vi "ControlKeithley2614_B.vi"() -> ()   [LabVIEW 2015]
panel:
  in  "GPIB Address":string="12"
  out "String":string
  in  "Record new values":bool
  out "Output Current (A)":dbl
  out "Output Voltage (V)":dbl
  out "Compliance limit (V)":dbl
  out "Current Range":u16(ring) items=["100 nA", "1 uA", "10 uA", "100 uA", "1 mA", "10 mA", "100 mA", "1 A"]
  out "Voltage Range":u16(ring) items=["200 mV", "2 V", "20 V", "200 V"]
  out "Current (sourse)":dbl
  out "Voltage (sourse)":dbl
  out "ComplianceIndicator":bool
  out "Compliance limit (A)":dbl
  out "Source Function":u16(ring)=1 items=["Current Source", "Voltage Source"]
  out "Sence Mode":u16(ring) items=["2-wire", "4-wire"]
  in  "ON/OFF channel":bool
  out "ON/OFF indicator":bool
  in  "error in (no error)":errorcluster
  out "error out":errorcluster
  # "Channel B"
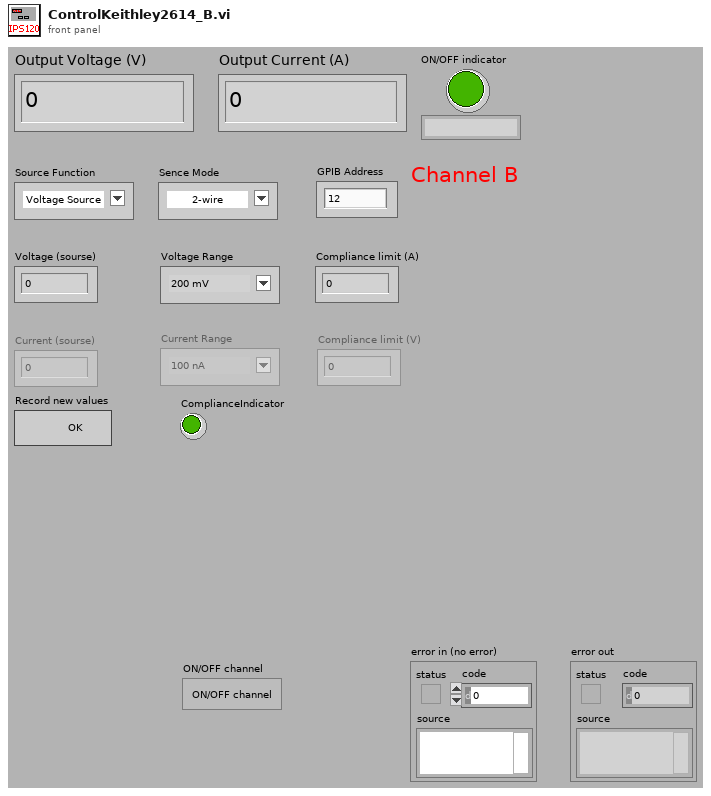
[diagram p1: front panel]
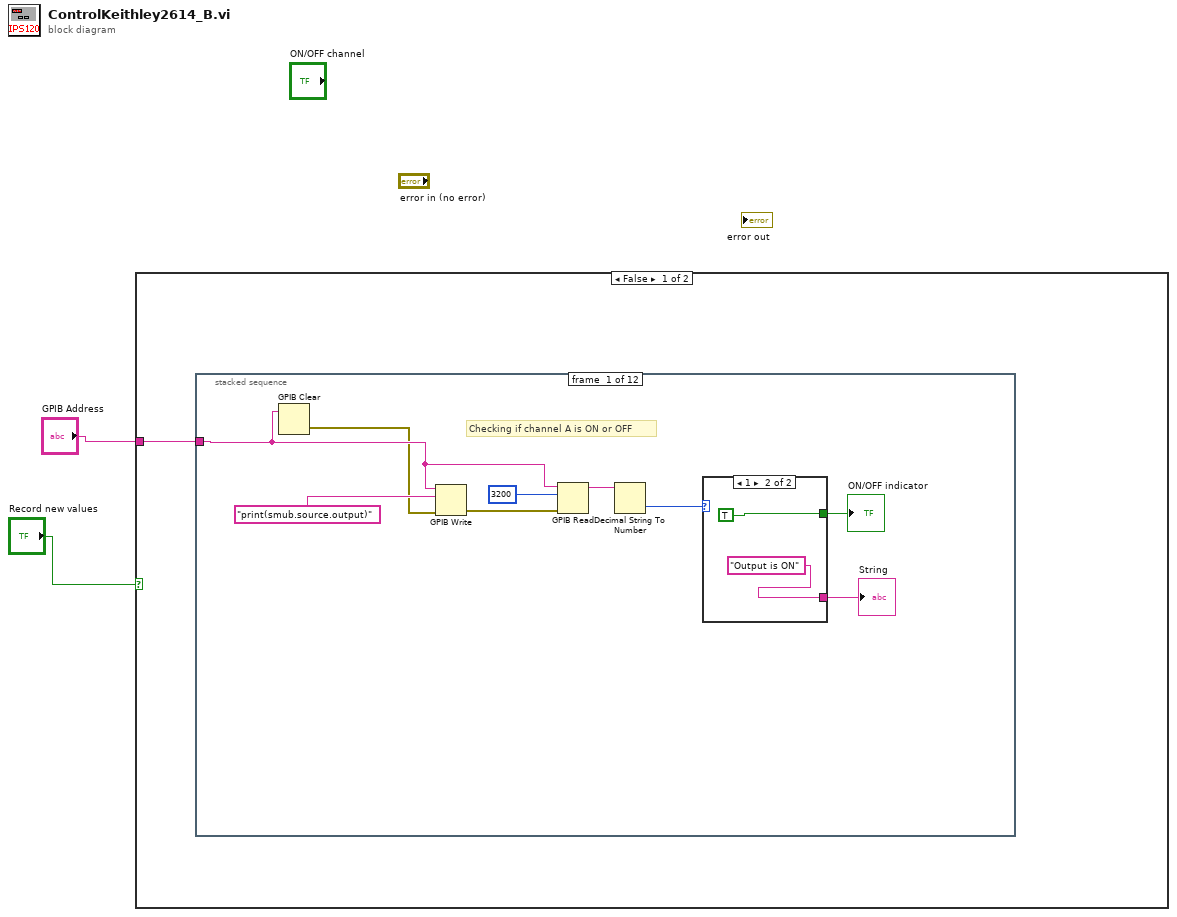
[diagram p0: block diagram]
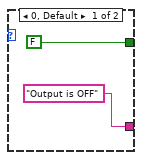
[diagram p2: hidden frame]
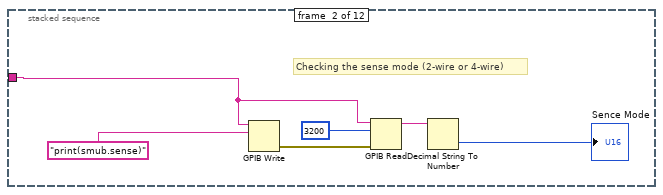
[diagram p3: hidden frame]
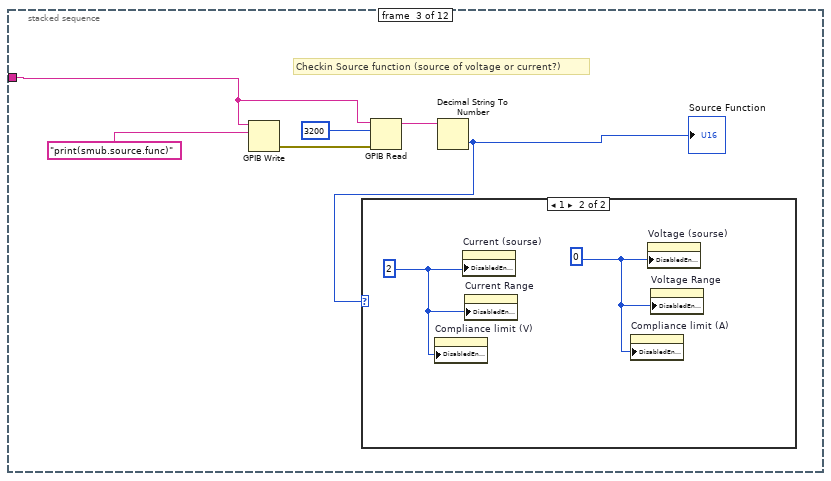
[diagram p4: hidden frame]
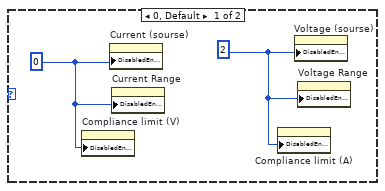
[diagram p5: hidden frame]
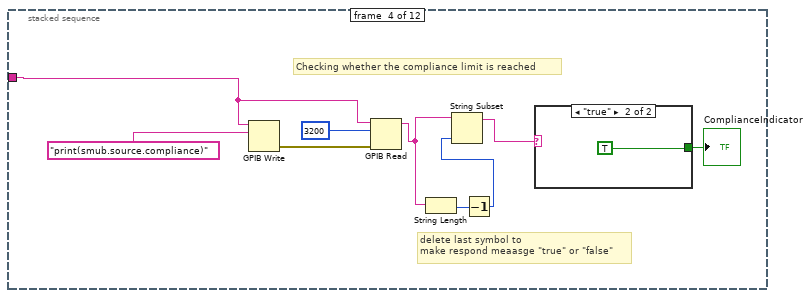
[diagram p6: hidden frame]
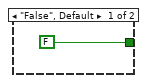
[diagram p7: hidden frame]
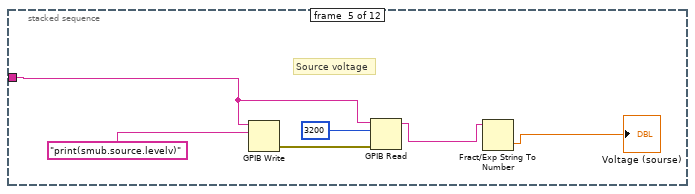
[diagram p8: hidden frame]
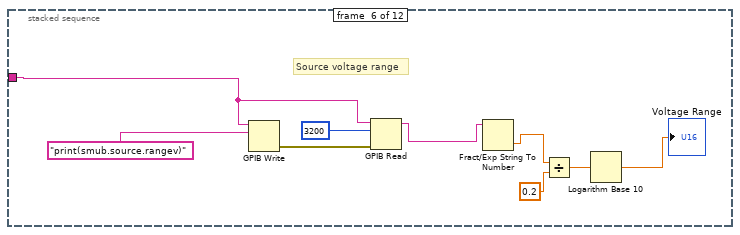
[diagram p9: hidden frame]
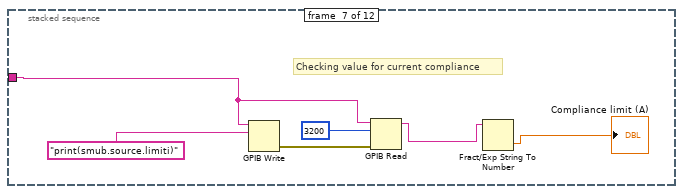
[diagram p10: hidden frame]
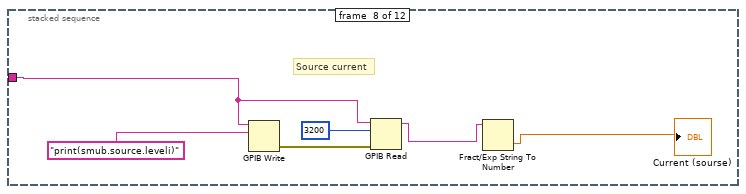
[diagram p11: hidden frame]
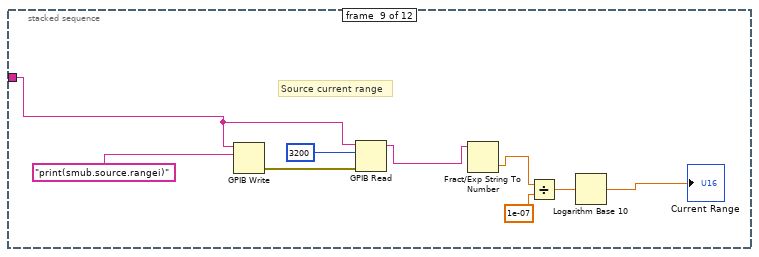
[diagram p12: hidden frame]
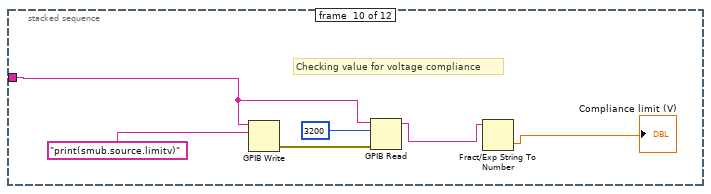
[diagram p13: hidden frame]
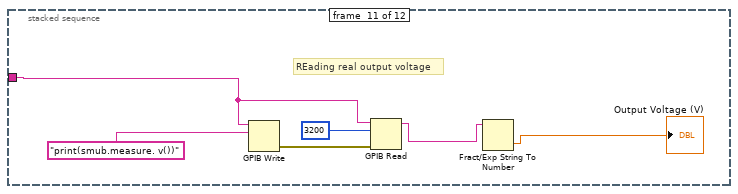
[diagram p14: hidden frame]
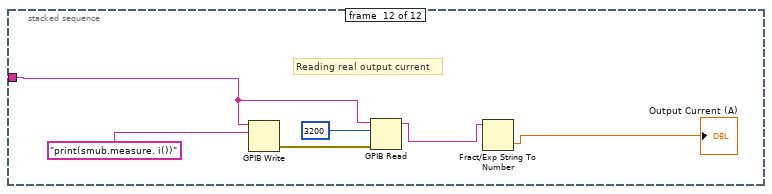
[diagram p15: hidden frame]
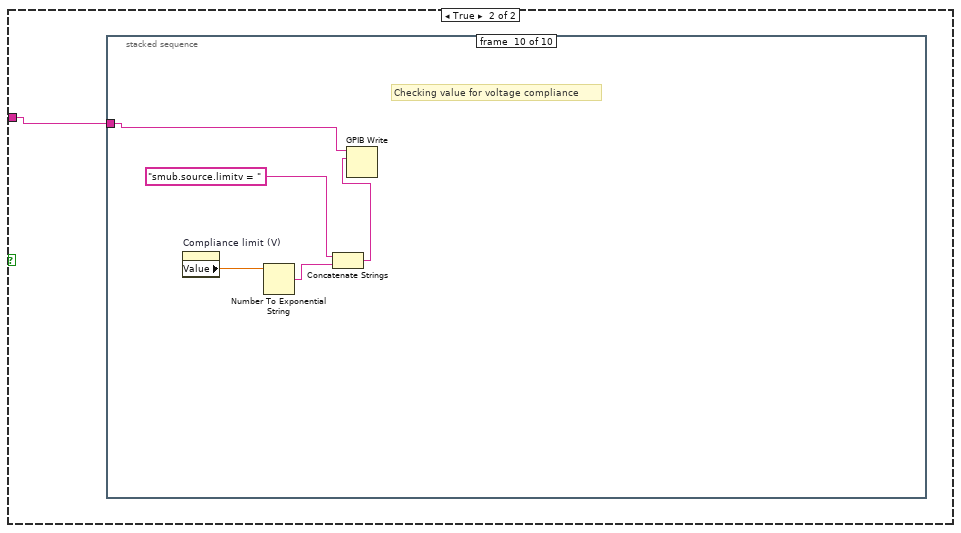
[diagram p16: hidden frame]
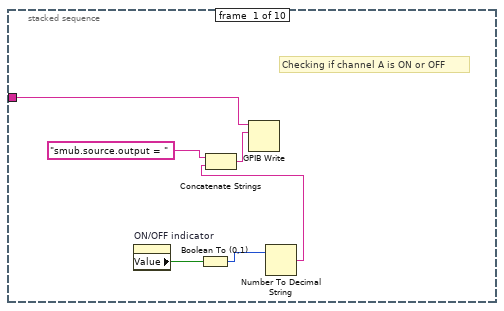
[diagram p17: hidden frame]
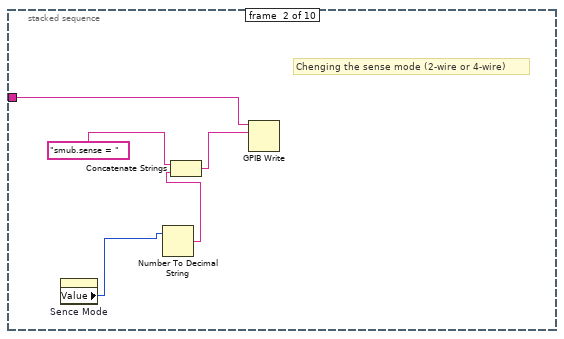
[diagram p18: hidden frame]
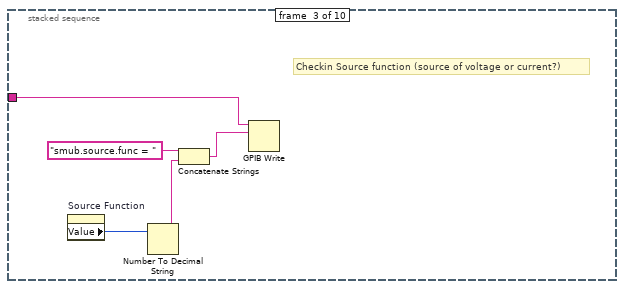
[diagram p19: hidden frame]
diagram:
  n1 = case shown="False" "Record new values" {
    tunnel: "GPIB Address" -> [w3 w98]
    frame False {
      n2 = stacked-sequence {
        tunnel: w3 -> [w5 w17 w23 w33 w44 w50 w59 w65 w71 w80 w86 w92]
        frame #0 {
          # "Checking if channel A is ON or OFF"
          n3 = GPIB Clear(3:w5) -> (0:w4:errorcluster)  [unwired: 1 in, 1 out]
          n4 = GPIB Write(0:w5, 1:"print(smub.source.output)", 3:w4) -> (6:w12:errorcluster)  [unwired: 2 in, 1 out]
          n5 = GPIB Read(0:w5, 1:3200, 3:w12) -> (5:w9:string)  [unwired: 2 in, 2 out]
          n6 = Decimal String To Number(string=w9) -> (number=w8:i32)  [unwired: 2 in, 1 out]
          n7 = case shown="1" w8 {
            tunnel: [FALSE TRUE] -> w7
            tunnel: ["Output is OFF" "Output is ON"] -> w6
            frame 0, Default {
            }
            frame 1 {
            }
          }
          "ON/OFF indicator" <- w7
          "String" <- w6
        }
        frame #1 {
          # "Checking the sense mode (2-wire or 4-wire)"
          n8 = GPIB Write(0:w17, 1:"print(smub.sense)") -> (6:w22:errorcluster)  [unwired: 3 in, 1 out]
          n9 = GPIB Read(0:w17, 1:3200, 3:w22) -> (5:w19:string)  [unwired: 2 in, 2 out]
          n10 = Decimal String To Number(string=w19) -> (number=→"Sence Mode":i32)  [unwired: 2 in, 1 out]
        }
        frame #2 {
          # "Checkin Source function (source of voltage or current?)"
          n11 = GPIB Write(0:w23, 1:"print(smub.source.func)") -> (6:w28:errorcluster)  [unwired: 3 in, 1 out]
          n12 = GPIB Read(0:w23, 1:3200, 3:w28) -> (5:w25:string)  [unwired: 2 in, 2 out]
          n13 = Decimal String To Number(string=w25) -> (number=w24:i32)  [unwired: 2 in, 1 out]
          "Source Function" <- w24
          n14 = case shown="1" w24 {
            frame 0, Default {
              w29 = 2
              w30 = 0
              n15 = property on="Compliance limit (V)" class="DigNum (strict)"("DisabledEnum"=w30) -> ()  [unwired: 2 in, 2 out]
              n16 = property on="Current (sourse)" class="DigNum (strict)"("DisabledEnum"=w30) -> ()  [unwired: 2 in, 2 out]
              n17 = property on="Current Range" class="Ring (strict)"("DisabledEnum"=w30) -> ()  [unwired: 2 in, 2 out]
              n18 = property on="Compliance limit (A)" class="DigNum (strict)"("DisabledEnum"=w29) -> ()  [unwired: 2 in, 2 out]
              n19 = property on="Voltage (sourse)" class="DigNum (strict)"("DisabledEnum"=w29) -> ()  [unwired: 2 in, 2 out]
              n20 = property on="Voltage Range" class="Ring (strict)"("DisabledEnum"=w29) -> ()  [unwired: 2 in, 2 out]
            }
            frame 1 {
              w31 = 0
              w32 = 2
              n21 = property on="Compliance limit (V)" class="DigNum (strict)"("DisabledEnum"=w32) -> ()  [unwired: 2 in, 2 out]
              n22 = property on="Current (sourse)" class="DigNum (strict)"("DisabledEnum"=w32) -> ()  [unwired: 2 in, 2 out]
              n23 = property on="Current Range" class="Ring (strict)"("DisabledEnum"=w32) -> ()  [unwired: 2 in, 2 out]
              n24 = property on="Compliance limit (A)" class="DigNum (strict)"("DisabledEnum"=w31) -> ()  [unwired: 2 in, 2 out]
              n25 = property on="Voltage (sourse)" class="DigNum (strict)"("DisabledEnum"=w31) -> ()  [unwired: 2 in, 2 out]
              n26 = property on="Voltage Range" class="Ring (strict)"("DisabledEnum"=w31) -> ()  [unwired: 2 in, 2 out]
            }
          }
        }
        frame #3 {
          # "delete last symbol to\nmake respond meaasge \"true\" or \"false\""
          # "Checking whether the compliance limit is reached"
          n27 = GPIB Write(0:w33, 1:"print(smub.source.compliance)") -> (6:w41:errorcluster)  [unwired: 3 in, 1 out]
          n28 = GPIB Read(0:w33, 1:3200, 3:w41) -> (5:w35:string)  [unwired: 2 in, 2 out]
          n29 = String Length(string=w35) -> (length=w37:i32)
          n30 = Decrement(x=w37) -> (x-1=w36:i32)
          n31 = String Subset(string=w35, length (rest)=w36) -> (substring=w34:string)  [unwired: 1 in]
          n32 = case shown="\"true\"" w34 {
            tunnel: [FALSE TRUE] -> w38
            frame "False", Default {
            }
            frame "true" {
            }
          }
          "ComplianceIndicator" <- w38
        }
        frame #4 {
          # "Source voltage"
          n33 = GPIB Write(0:w44, 1:"print(smub.source.levelv)") -> (6:w49:errorcluster)  [unwired: 3 in, 1 out]
          n34 = GPIB Read(0:w44, 1:3200, 3:w49) -> (5:w46:string)  [unwired: 2 in, 2 out]
          n35 = Fract/Exp String To Number(string=w46) -> (number=→"Voltage (sourse)":dbl)  [unwired: 3 in, 1 out]
        }
        frame #5 {
          # "Source voltage range"
          n36 = GPIB Write(0:w50, 1:"print(smub.source.rangev)") -> (6:w58:errorcluster)  [unwired: 3 in, 1 out]
          n37 = GPIB Read(0:w50, 1:3200, 3:w58) -> (5:w55:string)  [unwired: 2 in, 2 out]
          n38 = Fract/Exp String To Number(string=w55) -> (number=w53:dbl)  [unwired: 3 in, 1 out]
          n39 = Divide(x=w53, y=0.2) -> (x/y=w52:dbl)
          n40 = Logarithm Base 10(1:w52) -> (0:→"Voltage Range":dbl)
        }
        frame #6 {
          # "Checking value for current compliance"
          n41 = GPIB Write(0:w59, 1:"print(smub.source.limiti)") -> (6:w64:errorcluster)  [unwired: 3 in, 1 out]
          n42 = GPIB Read(0:w59, 1:3200, 3:w64) -> (5:w61:string)  [unwired: 2 in, 2 out]
          n43 = Fract/Exp String To Number(string=w61) -> (number=→"Compliance limit (A)":dbl)  [unwired: 3 in, 1 out]
        }
        frame #7 {
          # "Source current"
          n44 = GPIB Write(0:w65, 1:"print(smub.source.leveli)") -> (6:w70:errorcluster)  [unwired: 3 in, 1 out]
          n45 = GPIB Read(0:w65, 1:3200, 3:w70) -> (5:w67:string)  [unwired: 2 in, 2 out]
          n46 = Fract/Exp String To Number(string=w67) -> (number=→"Current (sourse)":dbl)  [unwired: 3 in, 1 out]
        }
        frame #8 {
          # "Source current range"
          n47 = GPIB Write(0:w71, 1:"print(smub.source.rangei)") -> (6:w79:errorcluster)  [unwired: 3 in, 1 out]
          n48 = GPIB Read(0:w71, 1:3200, 3:w79) -> (5:w76:string)  [unwired: 2 in, 2 out]
          n49 = Fract/Exp String To Number(string=w76) -> (number=w74:dbl)  [unwired: 3 in, 1 out]
          n50 = Divide(x=w74, y=1e-07) -> (x/y=w73:dbl)
          n51 = Logarithm Base 10(1:w73) -> (0:→"Current Range":dbl)
        }
        frame #9 {
          # "Checking value for voltage compliance"
          n52 = GPIB Write(0:w80, 1:"print(smub.source.limitv)") -> (6:w85:errorcluster)  [unwired: 3 in, 1 out]
          n53 = GPIB Read(0:w80, 1:3200, 3:w85) -> (5:w82:string)  [unwired: 2 in, 2 out]
          n54 = Fract/Exp String To Number(string=w82) -> (number=→"Compliance limit (V)":dbl)  [unwired: 3 in, 1 out]
        }
        frame #10 {
          # "REading real output voltage"
          n55 = GPIB Write(0:w86, 1:"print(smub.measure. v())") -> (6:w91:errorcluster)  [unwired: 3 in, 1 out]
          n56 = GPIB Read(0:w86, 1:3200, 3:w91) -> (5:w88:string)  [unwired: 2 in, 2 out]
          n57 = Fract/Exp String To Number(string=w88) -> (number=→"Output Voltage (V)":dbl)  [unwired: 3 in, 1 out]
        }
        frame #11 {
          # "Reading real output current"
          n58 = GPIB Write(0:w92, 1:"print(smub.measure. i())") -> (6:w97:errorcluster)  [unwired: 3 in, 1 out]
          n59 = GPIB Read(0:w92, 1:3200, 3:w97) -> (5:w94:string)  [unwired: 2 in, 2 out]
          n60 = Fract/Exp String To Number(string=w94) -> (number=→"Output Current (A)":dbl)  [unwired: 3 in, 1 out]
        }
      }
    }
    frame True {
      n61 = stacked-sequence {
        tunnel: w98 -> [w99 w105 w110 _ w115 w120 w128 w133 w138 w146]
        frame #0 {
          # "Checking if channel A is ON or OFF"
          n62 = property on="ON/OFF indicator" class="Bool (strict)"() -> ("Value"=w104:bool)  [unwired: 2 in, 2 out]
          n63 = Boolean To (0,1)(Boolean=w104) -> (0, 1=w103:i16)
          n64 = Number To Decimal String(number=w103) -> (decimal integer string=w101:string)  [unwired: 1 in]
          n65 = Concatenate Strings("smub.source.output = ", w101) -> (w100:string)
          n66 = GPIB Write(0:w99, 1:w100) -> ()  [unwired: 3 in, 2 out]
        }
        frame #1 {
          # "Chenging the sense mode (2-wire or 4-wire)"
          n67 = property on="Sence Mode" class="Ring (strict)"() -> ("Value"=w106:u16)  [unwired: 2 in, 2 out]
          n68 = Number To Decimal String(number=w106) -> (decimal integer string=w108:string)  [unwired: 1 in]
          n69 = Concatenate Strings("smub.sense = ", w108) -> (w107:string)
          n70 = GPIB Write(0:w105, 1:w107) -> ()  [unwired: 3 in, 2 out]
        }
        frame #2 {
          # "Checkin Source function (source of voltage or current?)"
          n71 = property on="Source Function" class="Ring (strict)"() -> ("Value"=w113:u16)  [unwired: 2 in, 2 out]
          n72 = Number To Decimal String(number=w113) -> (decimal integer string=w112:string)  [unwired: 1 in]
          n73 = Concatenate Strings("smub.source.func = ", w112) -> (w111:string)
          n74 = GPIB Write(0:w110, 1:w111) -> ()  [unwired: 3 in, 2 out]
        }
        frame #3 {
        }
        frame #4 {
          # "Source voltage"
          n75 = property on="Voltage (sourse)" class="DigNum (strict)"() -> ("Value"=w118:dbl)  [unwired: 2 in, 2 out]
          n76 = Number To Exponential String(number=w118) -> (E-format string=w117:string)  [unwired: 3 in]
          n77 = Concatenate Strings("smub.source.levelv = ", w117) -> (w116:string)
          n78 = GPIB Write(0:w115, 1:w116) -> ()  [unwired: 3 in, 2 out]
        }
        frame #5 {
          # "Source voltage range"
          n79 = property on="Voltage Range" class="Ring (strict)"() -> ("Value"=w127:u16)  [unwired: 2 in, 2 out]
          n80 = Power Of 10(x=w127) -> (10^x=w122:dbl)
          n81 = Multiply(x=w122, y=0.2) -> (x*y=w121:dbl)
          n82 = Number To Exponential String(number=w121) -> (E-format string=w126:string)  [unwired: 3 in]
          n83 = Concatenate Strings("smub.source.rangev = ", w126) -> (w124:string)
          n84 = GPIB Write(0:w120, 1:w124) -> ()  [unwired: 3 in, 2 out]
        }
        frame #6 {
          # "Checking value for current compliance"
          n85 = property on="Compliance limit (A)" class="DigNum (strict)"() -> ("Value"=w132:dbl)  [unwired: 2 in, 2 out]
          n86 = Number To Exponential String(number=w132) -> (E-format string=w131:string)  [unwired: 3 in]
          n87 = Concatenate Strings("smub.source.limiti = ", w131) -> (w129:string)
          n88 = GPIB Write(0:w128, 1:w129) -> ()  [unwired: 3 in, 2 out]
        }
        frame #7 {
          # "Source current"
          n89 = property on="Current (sourse)" class="DigNum (strict)"() -> ("Value"=w136:dbl)  [unwired: 2 in, 2 out]
          n90 = Number To Exponential String(number=w136) -> (E-format string=w137:string)  [unwired: 3 in]
          n91 = Concatenate Strings("smub.source.leveli = ", w137) -> (w134:string)
          n92 = GPIB Write(0:w133, 1:w134) -> ()  [unwired: 3 in, 2 out]
        }
        frame #8 {
          # "Source current range"
          n93 = property on="Current Range" class="Ring (strict)"() -> ("Value"=w145:u16)  [unwired: 2 in, 2 out]
          n94 = Power Of 10(x=w145) -> (10^x=w144:dbl)
          n95 = Multiply(x=w144, y=1e-07) -> (x*y=w142:dbl)
          n96 = Number To Exponential String(number=w142) -> (E-format string=w141:string)  [unwired: 3 in]
          n97 = Concatenate Strings("smub.source.rangei = ", w141) -> (w139:string)
          n98 = GPIB Write(0:w138, 1:w139) -> ()  [unwired: 3 in, 2 out]
        }
        frame #9 {
          # "Checking value for voltage compliance"
          n99 = property on="Compliance limit (V)" class="DigNum (strict)"() -> ("Value"=w148:dbl)  [unwired: 2 in, 2 out]
          n100 = Number To Exponential String(number=w148) -> (E-format string=w147:string)  [unwired: 3 in]
          n101 = Concatenate Strings("smub.source.limitv = ", w147) -> (w149:string)
          n102 = GPIB Write(0:w146, 1:w149) -> ()  [unwired: 3 in, 2 out]
        }
      }
    }
  }
